vi "temp read.vi"() -> ()   [LabVIEW 2021]
uses:
  <vilib>/Instr/_visa.llb/VISA Configure Serial Port (Instr).vi
panel:
  out "Waveform Chart":dbl[](graph)
  in  "Boolean":bool
  in  "Stop Button":bool
  out "array":dbl[](array[numeric])
  out "String":string
  in  "Numeric":u32
  in  "VISA resource name":refnum<visa-resource-name>
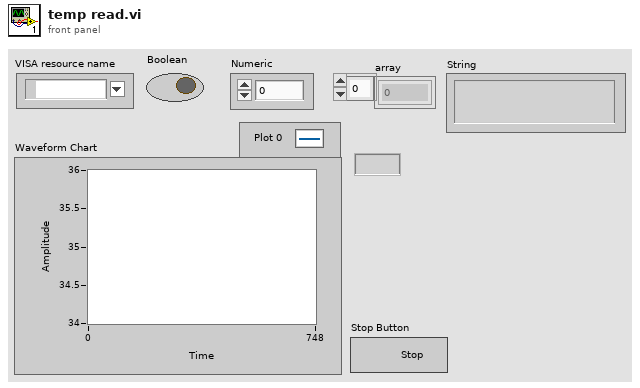
[diagram p1: front panel]
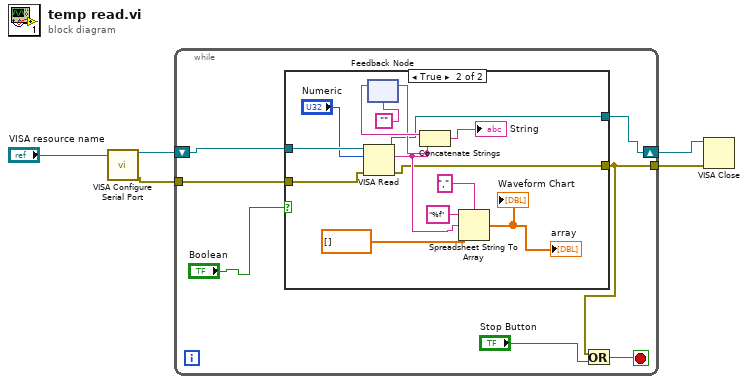
[diagram p0: block diagram]
diagram:
  n1 = call-poly "VISA Configure Serial Port"("VISA resource name"="VISA resource name") -> ("VISA resource name out"=w4:refnum<visa-resource-name>, "error out"=w3:errorcluster)  [unwired: 13 in]
  n2 = while {
    shift-right: [w10] -> w2
    shift-left: w4 -> [w12]
    tunnel: w3 -> [w11]
    tunnel: [w8] -> w1
    stop <- w9 stop-if-true
    n3 = case shown="True" "Boolean" {
      tunnel: w12 -> [w14 w27]
      tunnel: w11 -> [w13 w26]
      tunnel: [w14 w17] -> w10
      tunnel: [w13 w16] -> w8
      frame False {
      }
      frame True {
        n4 = VISA Read(VISA resource name=w27, byte count="Numeric", error in (no error)=w26) -> (VISA resource name out=w17:refnum<visa-resource-name>, read buffer=w19:string, error out=w16:errorcluster)  [unwired: 1 out]
        n5 = feedback-in #1(w19) -> ()
        n6 = feedback #1("") -> (w23:string)
        n7 = Concatenate Strings(w23, w19) -> (→"String":string)
        n8 = Spreadsheet String To Array(delimiter (Tab)=",", format string="%f", spreadsheet string=w19, array type (2D Dbl)=dbl[] []) -> (array=→"array" →"Waveform Chart":dbl[])
      }
    }
    n9 = Or(x=w8, y="Stop Button") -> (x .or. y?=w9:bool)
  }
  n10 = VISA Close(VISA resource name=w2, error in (no error)=w1) -> ()  [unwired: 1 out]
